vi "SQL_configuration_update.vi"(11 "表格控件":string[][](table)) -> (3 "error out":errorcluster)   [LabVIEW 2014]
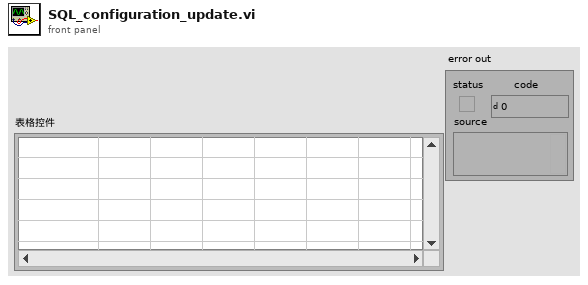
[diagram p1: front panel]
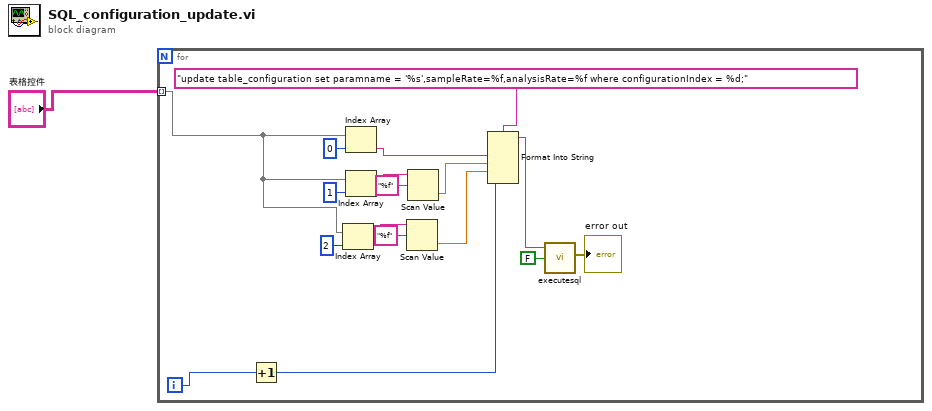
[diagram p0: block diagram]
diagram:
  n1 = for {
    tunnel: "表格控件" -> [w7] mode=indexing
    i -> [w4]
    n2 = Increment(x=w4) -> (x+1=w3:i32)
    n3 = Index Array(array=w7, index=2 ("索引")) -> (element=w9:string)
    n4 = Index Array(array=w7, index=0 ("索引")) -> (element=w16:string)
    n5 = Index Array(array=w7, index=1 ("索引")) -> (element=w14:string)
    n6 = Scan Value(string=w9, format string="%f" ("格式字符串")) -> (value=w8:dbl)  [unwired: 1 in, 1 out]
    n7 = Scan Value(string=w14, format string="%f" ("格式字符串")) -> (value=w13:dbl)  [unwired: 1 in, 1 out]
    n8 = Format Into String(format string="update table_configuration set paramname = '%s',sampleRate=%f,analysisRate=%f where configurationIndex = %d;", w16, w13, w8, w3) -> (resulting string=w12:string)  [unwired: 2 in, 1 out]
    n9 = call "executesql.vi"("Return Data (T)"=FALSE, "Command Text"=w12) -> ("error out"=→"error out":errorcluster)  [unwired: 5 in, 1 out]
  }
